vi "Load Children By Config.vi"(0 "ActorMeter in":refnum<class "ActorMeter.lvclass">, 6 "error in (no error)":errorcluster) -> (20 "ActorMeter out":refnum<class "ActorMeter.lvclass">, 21 "ParameterDevice.lvclass":refnum<class "ParameterDevice.lvclass">, 22 "ReadoutDevice.lvclass":refnum<class "ReadoutDevice.lvclass">, 23 "AbstractProcessor.lvclass":refnum<class "AbstractProcessor.lvclass">, 24 "AbstractCollector.lvclass":refnum<class "AbstractCollector.lvclass">, 25 "AbstractExtractor.lvclass":refnum<class "AbstractExtractor.lvclass">, 26 "error out":errorcluster)   [LabVIEW 2014, in "ActorMeter.lvclass"]
uses:
  ActorMeter.lvclass
  Hardware/ReadoutDevice/ReadoutDevice.lvclass
  Hardware/ParameterDevice/ParameterDevice.lvclass
  Collector/AbstractCollector/AbstractCollector.lvclass
  Processor/AbstractProcessor/AbstractProcessor.lvclass
  Extractor/AbstractExtractor/AbstractExtractor.lvclass
  ActorMeter.lvclass/ActorMeter.ctl
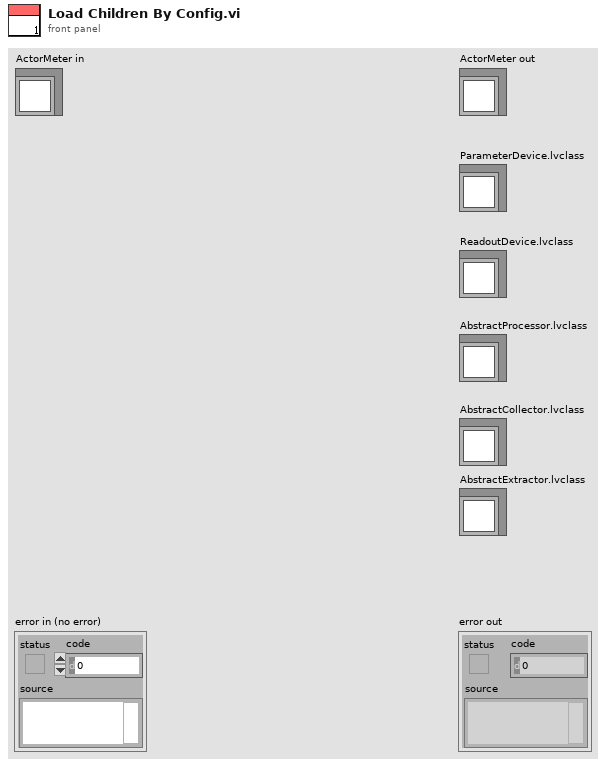
[diagram p1: front panel]
types:
  T1 = typedef "Registry.ctl" = cluster{"type":string, "elements":cluster{"name":string, "path":string}[]}[]
  T2 = typedef "Configuration.ctl" = cluster{"type":string, "name":string}[]
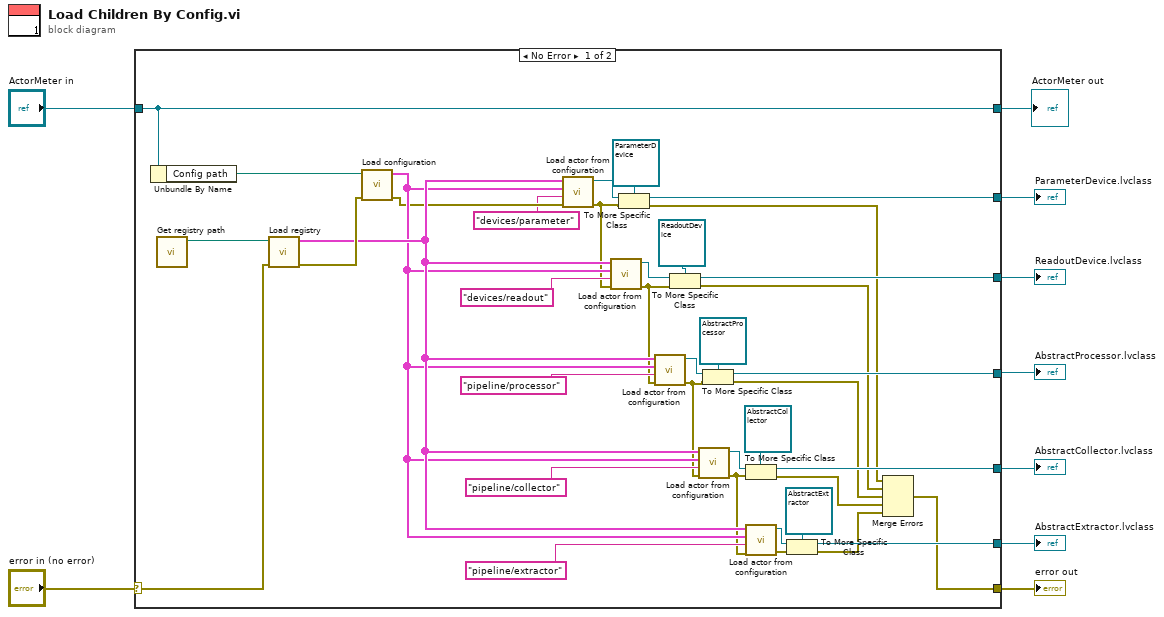
[diagram p0: block diagram]
diagram:
  n1 = case shown="No Error" "error in (no error)" {
    selector: "error in (no error)" -> [w11 w50]
    tunnel: [w10 w50] -> w8
    tunnel: [w48 w49] -> w6
    tunnel: "ActorMeter in" -> [w48 w49]
    tunnel: [w21 _] -> w1
    tunnel: [w20 _] -> w2
    tunnel: [w19 _] -> w3
    tunnel: [w18 _] -> w4
    tunnel: [w17 _] -> w5
    frame No Error {
      n2 = Unbundle By Name(w48) -> ("Config path"=w46:path)
      n3 = call "Get registry path.vi"() -> ("Registry path"=w47:path)  [unwired: 11 in]
      n4 = call "Load registry.vi"("error in"=w11, "Path"=w47) -> ("error out"=w45:errorcluster, "Registry"=w44:T1)  [unwired: 8 in]
      n5 = call "Load configuration.vi"("error in"=w45, "Path"=w46) -> ("error out"=w42:errorcluster, "Configuration"=w43:T2)  [unwired: 8 in]
      n6 = call "Load actor from configuration.vi"("error in (no error)"=w42, "Type"="devices/parameter", "Configuration"=w43, "Registry"=w44) -> ("error out"=w36:errorcluster, "Actor"=w34:refnum<class "Actor.lvclass">)  [unwired: 6 in]
      n7 = call "Load actor from configuration.vi"("error in (no error)"=w36, "Type"="devices/readout", "Configuration"=w43, "Registry"=w44) -> ("error out"=w33:errorcluster, "Actor"=w31:refnum<class "Actor.lvclass">)  [unwired: 6 in]
      n8 = To More Specific Class(target class=refnum<class "ParameterDevice.lvclass"> refnum ("ParameterDevice.lvclass"), reference=w34, error in=w36) -> (specific class reference=w21:refnum<class "ParameterDevice.lvclass">, error out=w16:errorcluster)
      n9 = call "Load actor from configuration.vi"("error in (no error)"=w33, "Type"="pipeline/processor", "Configuration"=w43, "Registry"=w44) -> ("error out"=w28:errorcluster, "Actor"=w27:refnum<class "Actor.lvclass">)  [unwired: 6 in]
      n10 = To More Specific Class(target class=refnum<class "ReadoutDevice.lvclass"> refnum ("ReadoutDevice.lvclass"), reference=w31, error in=w33) -> (specific class reference=w20:refnum<class "ReadoutDevice.lvclass">, error out=w15:errorcluster)
      n11 = call "Load actor from configuration.vi"("error in (no error)"=w28, "Type"="pipeline/collector", "Configuration"=w43, "Registry"=w44) -> ("error out"=w29:errorcluster, "Actor"=w26:refnum<class "Actor.lvclass">)  [unwired: 6 in]
      n12 = To More Specific Class(target class=refnum<class "AbstractProcessor.lvclass"> refnum ("AbstractProcessor.lvclass"), reference=w27, error in=w28) -> (specific class reference=w19:refnum<class "AbstractProcessor.lvclass">, error out=w14:errorcluster)
      n13 = To More Specific Class(target class=refnum<class "AbstractCollector.lvclass"> refnum ("AbstractCollector.lvclass"), reference=w26, error in=w29) -> (specific class reference=w18:refnum<class "AbstractCollector.lvclass">, error out=w13:errorcluster)
      n14 = call "Load actor from configuration.vi"("error in (no error)"=w29, "Type"="pipeline/extractor", "Configuration"=w43, "Registry"=w44) -> ("error out"=w30:errorcluster, "Actor"=w22:refnum<class "Actor.lvclass">)  [unwired: 6 in]
      n15 = To More Specific Class(target class=refnum<class "AbstractExtractor.lvclass"> refnum ("AbstractExtractor.lvclass"), reference=w22, error in=w30) -> (specific class reference=w17:refnum<class "AbstractExtractor.lvclass">, error out=w12:errorcluster)
      n16 = Merge Errors(w16, w15, w14, w13, w12) -> (w10:errorcluster)
    }
    frame Error {
    }
  }
  "error out" <- w8
  "ActorMeter out" <- w6
  "AbstractExtractor.lvclass" <- w5
  "AbstractCollector.lvclass" <- w4
  "AbstractProcessor.lvclass" <- w3
  "ReadoutDevice.lvclass" <- w2
  "ParameterDevice.lvclass" <- w1
